vi "midiOutSustainPedal.vi"(8 "error in":errorcluster, 10 "value (0-127)":i32, 11 "midi in":refnum<class "midi.lvclass">) -> (0 "error out":errorcluster, 3 "midi out":refnum<class "midi.lvclass">)   [LabVIEW 2020, in "midi.lvclass"]
uses:
  midi.lvclass
  midichannel.get.vi
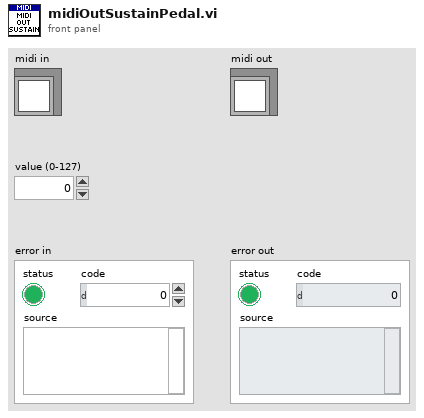
[diagram p1: front panel]
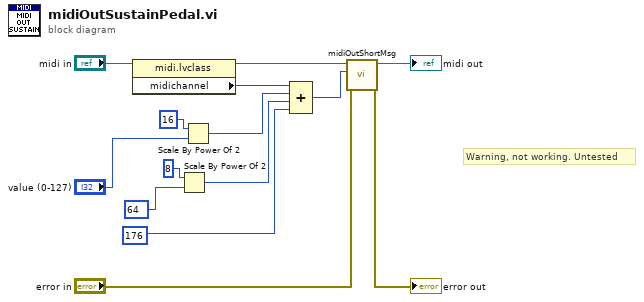
[diagram p0: block diagram]
diagram:
  # "Warning, not working. Untested"
  n1 = property class="midi.lvclass"(reference="midi in") -> (reference out=w6:refnum<class "midi.lvclass">, "midichannel"=w5:u64)  [unwired: 1 in, 1 out]
  n2 = Scale By Power Of 2(n=8, x=u8 64 ("Message")) -> (x*2^n=w14:u8)
  n3 = Scale By Power Of 2(n=i16 16, x="value (0-127)") -> (x*2^n=w13:i32)
  n4 = Compound Arithmetic op=ADD(w5, w13, w14, u8 176 ("Message")) -> (w1:u64)
  n5 = call "midiOutShortMsg.vi"("error in"="error in", "data"=w1, "midi in"=w6) -> ("error out"=→"error out":errorcluster, "midi out"=→"midi out":refnum<class "midi.lvclass">)  [unwired: 7 in]
